vi "parse_distance.vi"(8 "error in":errorcluster, 11 "msg in":string) -> (0 "error out":errorcluster, 2 "distance":cluster{"Left":dbl, "Middle":dbl, "Right":dbl}, 3 "msg out":string)   [LabVIEW 2016]
uses:
  <userlib>/ROS for LabVIEW Software/ROS/MessageParsing/std_msgs/subs/parse_float64_scalar.vi
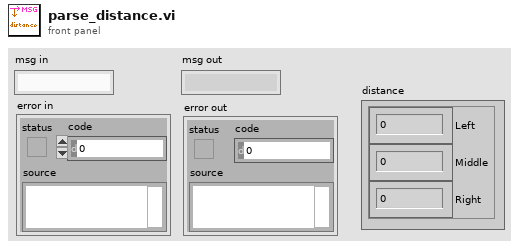
[diagram p1: front panel]
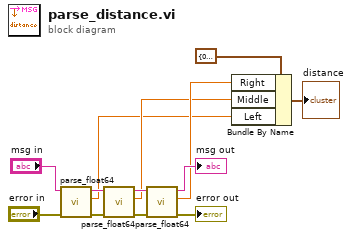
[diagram p0: block diagram]
diagram:
  n1 = call-poly <userlib>:"parse_float64.vi"("error in"="error in", "msg in"="msg in") -> ("error out"=w8:errorcluster, "number"=w1:dbl, "msg out"=w12:string)  [unwired: 3 in]
  n2 = call-poly <userlib>:"parse_float64.vi"("error in"=w8, "msg in"=w12) -> ("error out"=w7:errorcluster, "number"=w2:dbl, "msg out"=w11:string)  [unwired: 3 in]
  n3 = call-poly <userlib>:"parse_float64.vi"("error in"=w7, "msg in"=w11) -> ("error out"=→"error out":errorcluster, "number"=w3:dbl, "msg out"=→"msg out":string)  [unwired: 3 in]
  n4 = Bundle By Name(cluster=cluster{"Left":dbl, "Middle":dbl, "Right":dbl} {"Left"=0.0, "Middle"=0.0, "Right"=0.0}, "Right"=w3, "Middle"=w2, "Left"=w1) -> (→"distance":cluster{"Left":dbl, "Middle":dbl, "Right":dbl})
